vi "gauss.vi"(1 "X":dbl, 2 "amplitude":dbl, 3 "center":dbl, 4 "std. dev.":dbl) -> (0 "y":dbl)   [LabVIEW 2020]
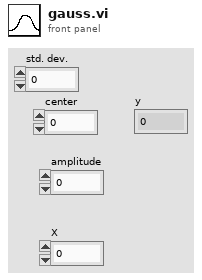
[diagram p1: front panel]
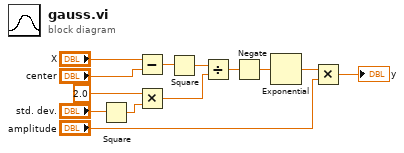
[diagram p0: block diagram]
diagram:
  n1 = Square(x="std. dev.") -> (x^2=w2:dbl)
  n2 = Subtract(x="X", y="center") -> (x-y=w10:dbl)
  n3 = Multiply(x=2.0, y=w2) -> (x*y=w6:dbl)
  n4 = Square(x=w10) -> (x^2=w9:dbl)
  n5 = Divide(x=w9, y=w6) -> (x/y=w5:dbl)
  n6 = Negate(x=w5) -> (-x=w13:dbl)
  n7 = Exponential(1:w13) -> (0:w7:dbl)
  n8 = Multiply(x=w7, y="amplitude") -> (x*y=→"y":dbl)
